vi "Refresh Data to Sysdef Data.vi"(8 "error in":errorcluster, 10 "Refresh Port":T1[](array[typedef])) -> (0 "error out":errorcluster, 2 "Refresh Sysdef":T5[](array[typedef]))   [LabVIEW 2020, in "Communication Bus Template System Explorer.lvlib" / "Implementation.lvlib"]
uses:
  Implementation.lvlib
  Types/Refresh For Sysdef.ctl
  Types/Frame.ctl
  Types/Signal.ctl
  Types/ECU.ctl
  Types/Refresh Port.ctl
  Types/Refresh Frame.ctl
  Types/Refresh Signal.ctl
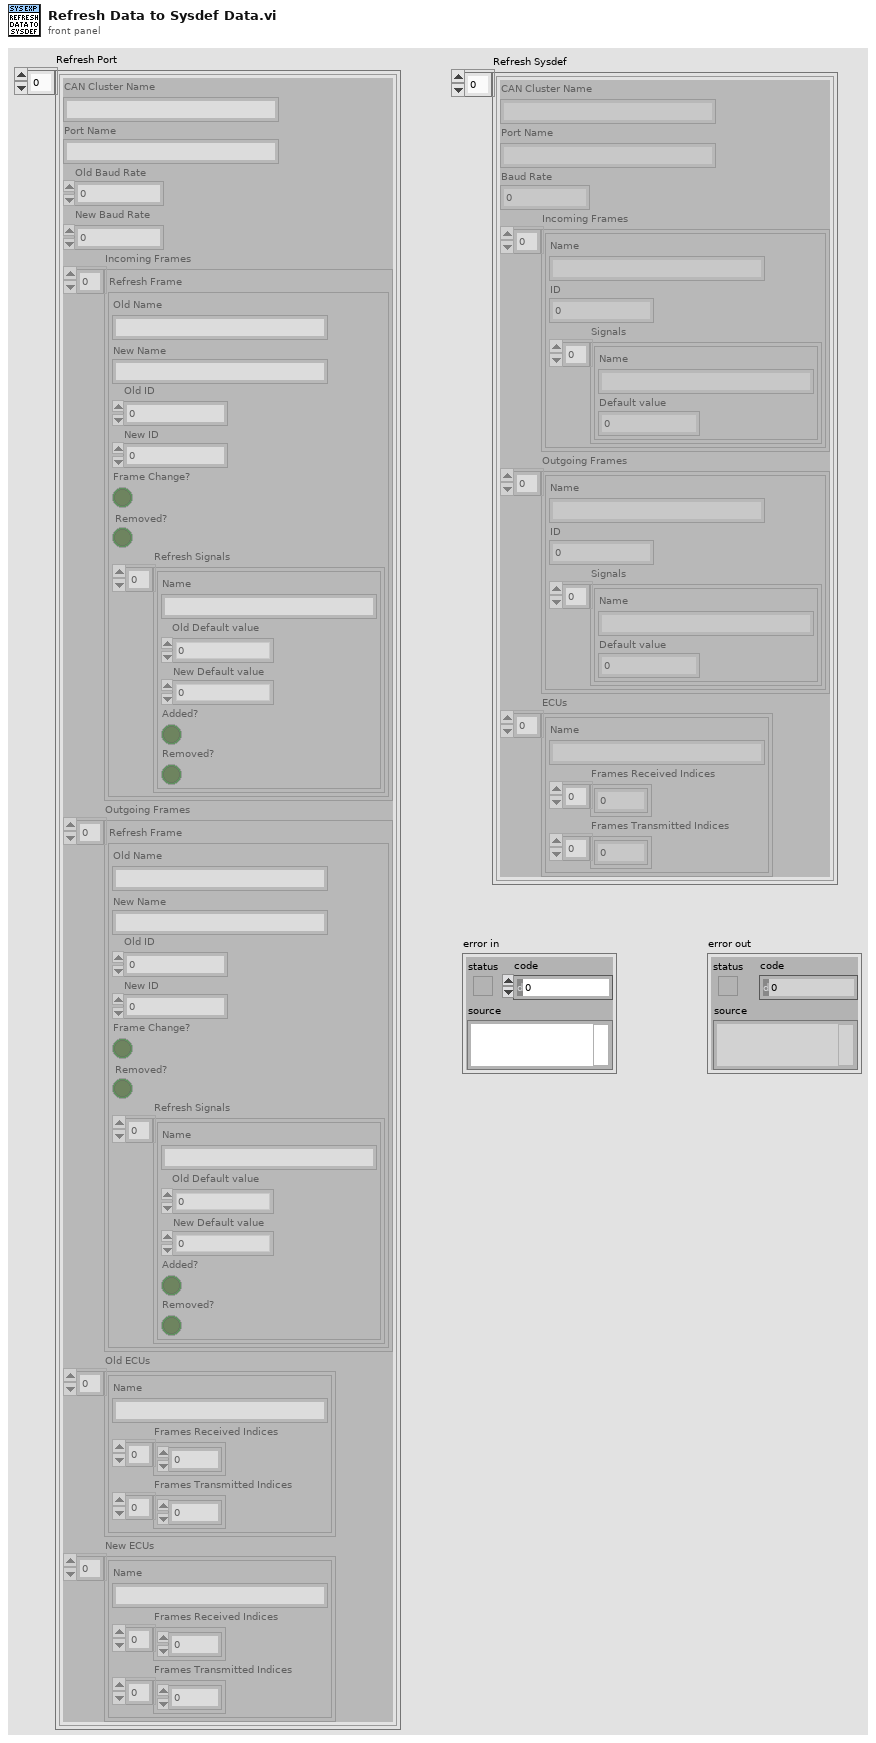
[diagram p1: front panel]
types:
  T1 = typedef "Communication Bus Template System Explorer.lvlib/Implementation.lvlib/Refresh Port.ctl" = cluster{"CAN Cluster Name":string, "Port Name":string, "Old Baud Rate":u64, "New Baud Rate":u64, "Incoming Frames":T2[], "Outgoing Frames":T2[], "Old ECUs":T4[], "New ECUs":T4[]}
  T2 = typedef "Communication Bus Template System Explorer.lvlib/Implementation.lvlib/Refresh Frame.ctl" = cluster{"Old Name":string, "New Name":string, "Old ID":u32, "New ID":u32, "Frame Change?":bool, "Removed?":bool, "Refresh Signals":T3[]}
  T3 = typedef "Communication Bus Template System Explorer.lvlib/Implementation.lvlib/Refresh Signal.ctl" = cluster{"Name":string, "Old Default value":dbl, "New Default value":dbl, "Added?":bool, "Removed?":bool}
  T4 = typedef "Communication Bus Template System Explorer.lvlib/Implementation.lvlib/ECU.ctl" = cluster{"Name":string, "Frames Received Indices":u32[], "Frames Transmitted Indices":u32[]}
  T5 = typedef "Communication Bus Template System Explorer.lvlib/Implementation.lvlib/Refresh For Sysdef.ctl" = cluster{"CAN Cluster Name":string, "Port Name":string, "Baud Rate":u64, "Incoming Frames":T6[], "Outgoing Frames":T6[], "ECUs":T4[]}
  T6 = typedef "Communication Bus Template System Explorer.lvlib/Implementation.lvlib/Frame.ctl" = cluster{"Name":string, "ID":u32, "Signals":T7[]}
  T7 = typedef "Communication Bus Template System Explorer.lvlib/Implementation.lvlib/Signal.ctl" = cluster{"Name":string, "Default value":dbl}
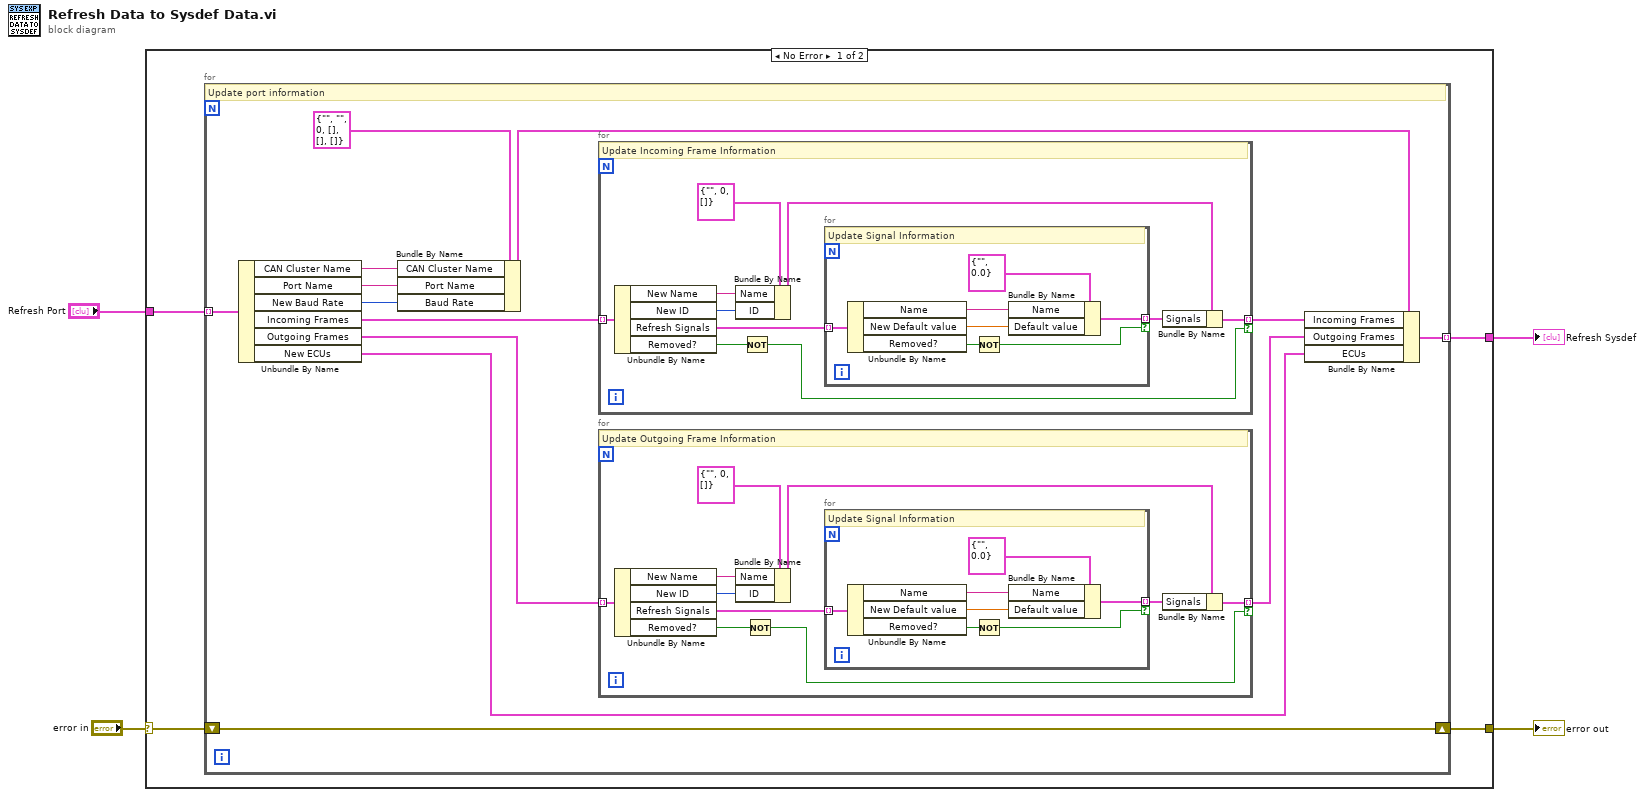
[diagram p0: block diagram]
diagram:
  n1 = case shown="No Error" "error in" {
    selector: "error in" -> [w8 w56]
    tunnel: [w5 _] -> w4
    tunnel: [w7 w56] -> w2
    tunnel: "Refresh Port" -> [w6 _]
    frame No Error {
      n2 = for {
        shift-right: [w21] -> w7
        shift-left: w8 -> [w21]
        tunnel: w6 -> [w16] mode=indexing
        tunnel: [w10] -> w5 mode=indexing
        # "Update port information"
        n3 = Unbundle By Name(w16) -> ("CAN Cluster Name"=w19:string, "Port Name"=w18:string, "New Baud Rate"=w17:u64, "Incoming Frames"=w15:T2[], "Outgoing Frames"=w12:T2[], "New ECUs"=w9:T4[])
        n4 = Bundle By Name(cluster=T5 {"CAN Cluster Name"="", "Port Name"="", "Baud Rate"=0, "Incoming Frames"=[], "Outgoing Frames"=[], "ECUs"=[]} ("CAN Cluster"), "CAN Cluster Name"=w19, "Port Name"=w18, "Baud Rate"=w17) -> (w14:T5)
        n5 = for {
          tunnel: w15 -> [w47] mode=indexing
          tunnel: [w41] -> w13 mode=indexing if=w39
          # "Update Incoming Frame Information"
          n6 = Unbundle By Name(w47) -> ("New Name"=w46:string, "New ID"=w45:u32, "Refresh Signals"=w44:T3[], "Removed?"=w40:bool)
          n7 = Bundle By Name(cluster=T6 {"Name"="", "ID"=0, "Signals"=[]} ("Frame"), "Name"=w46, "ID"=w45) -> (w43:T6)
          n8 = Not(x=w40) -> (.not. x?=w39:bool)
          n9 = for {
            tunnel: w44 -> [w55] mode=indexing
            tunnel: [w53] -> w42 mode=indexing if=w49
            # "Update Signal Information"
            n10 = Unbundle By Name(w55) -> ("Name"=w52:string, "New Default value"=w51:dbl, "Removed?"=w50:bool)
            n11 = Not(x=w50) -> (.not. x?=w49:bool)
            n12 = Bundle By Name(cluster=T7 {"Name"="", "Default value"=0.0} ("Signal"), "Name"=w52, "Default value"=w51) -> (w53:T7)
          }
          n13 = Bundle By Name(cluster=w43, "Signals"=w42) -> (w41:T6)
        }
        n14 = for {
          tunnel: w12 -> [w30] mode=indexing
          tunnel: [w24] -> w11 mode=indexing if=w22
          # "Update Outgoing Frame Information"
          n15 = Unbundle By Name(w30) -> ("New Name"=w29:string, "New ID"=w28:u32, "Refresh Signals"=w27:T3[], "Removed?"=w23:bool)
          n16 = Bundle By Name(cluster=T6 {"Name"="", "ID"=0, "Signals"=[]} ("Frame"), "Name"=w29, "ID"=w28) -> (w26:T6)
          n17 = Not(x=w23) -> (.not. x?=w22:bool)
          n18 = for {
            tunnel: w27 -> [w38] mode=indexing
            tunnel: [w36] -> w25 mode=indexing if=w32
            # "Update Signal Information"
            n19 = Unbundle By Name(w38) -> ("Name"=w35:string, "New Default value"=w34:dbl, "Removed?"=w33:bool)
            n20 = Not(x=w33) -> (.not. x?=w32:bool)
            n21 = Bundle By Name(cluster=T7 {"Name"="", "Default value"=0.0} ("Signal"), "Name"=w35, "Default value"=w34) -> (w36:T7)
          }
          n22 = Bundle By Name(cluster=w26, "Signals"=w25) -> (w24:T6)
        }
        n23 = Bundle By Name(cluster=w14, "Incoming Frames"=w13, "Outgoing Frames"=w11, "ECUs"=w9) -> (w10:T5)
      }
    }
    frame Error {
    }
  }
  "error out" <- w2
  "Refresh Sysdef" <- w4
